vi "Generate IMEI Report.vi"(6 "IMEI":string, 7 "Day":string, 8 "Daily Expected Tx % (IMEI Match):":string, 9 "% Good Tx. (IMEI Match)":string, 10 "Daily Tx (IMEI Match)":string, 11 "Daily Missed Tx (IMEI Match)":string) -> (3 "Report":string)   [LabVIEW 2014]
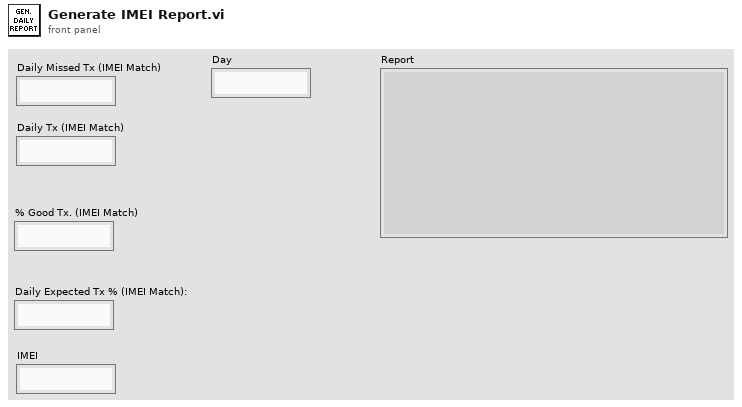
[diagram p1: front panel]
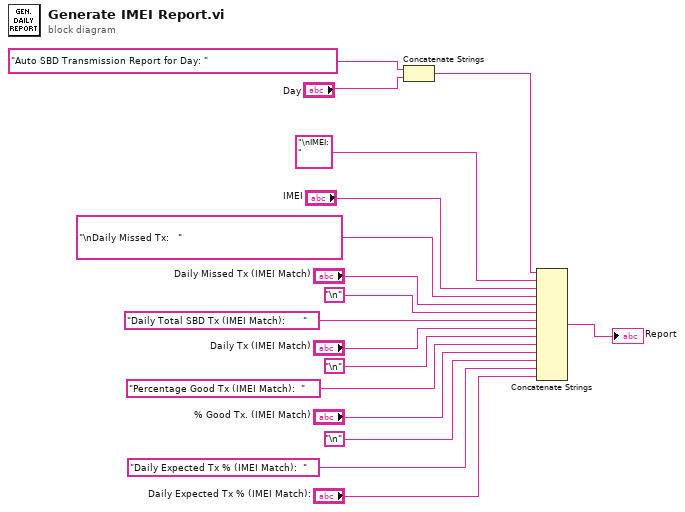
[diagram p0: block diagram]
diagram:
  n1 = Concatenate Strings("Auto SBD Transmission Report for Day: " ("string"), "Day") -> (w4:string)
  n2 = Concatenate Strings(w4, "\nIMEI: " ("string"), "IMEI", "\nDaily Missed Tx:   " ("string"), "Daily Missed Tx (IMEI Match)", "\n", "Daily Total SBD Tx (IMEI Match):      " ("string"), "Daily Tx (IMEI Match)", "\n", "Percentage Good Tx (IMEI Match):  " ("string"), "% Good Tx. (IMEI Match)", "\n", "Daily Expected Tx % (IMEI Match):  " ("string"), "Daily Expected Tx % (IMEI Match):") -> (→"Report":string)
